vi "Write to File.vi"(8 "error in (no error)":errorcluster, 10 "INI Ref":T1, 11 "Keyboard Macro in":refnum<class "Keyboard Macro.lvclass">) -> (0 "error out":errorcluster, 2 "INI Ref out":T1, 3 "Keyboard Macro out":refnum<class "Keyboard Macro.lvclass">)   [LabVIEW 2020, in "MacroAssert.lvlib" / "Keyboard Macro.lvclass"]
uses:
  Keyboard Macro.lvclass
  Keyboard Macro.lvclass/Keyboard Macro.ctl
  Macro Step/Macro Step.lvclass
  MacroAssert.lvlib
  <vilib>/Utility/config.llb/NI_LVConfig.lvlib
  <vilib>/Utility/config.llb/Write Key (String).vi
  <vilib>/Utility/config.llb/Write Key (Boolean).vi
  <vilib>/Utility/config.llb/Config Data RefNum.ctl
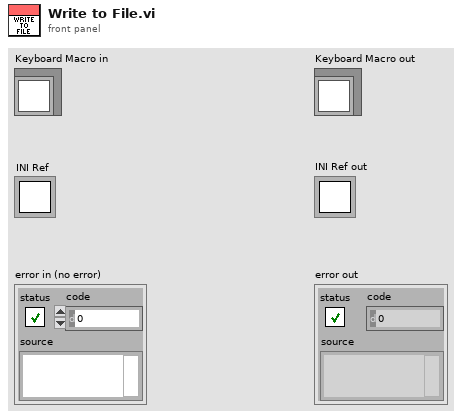
[diagram p1: front panel]
types:
  T1 = typedef "NI_LVConfig.lvlib/Config Data RefNum.ctl" = refnum<k1>
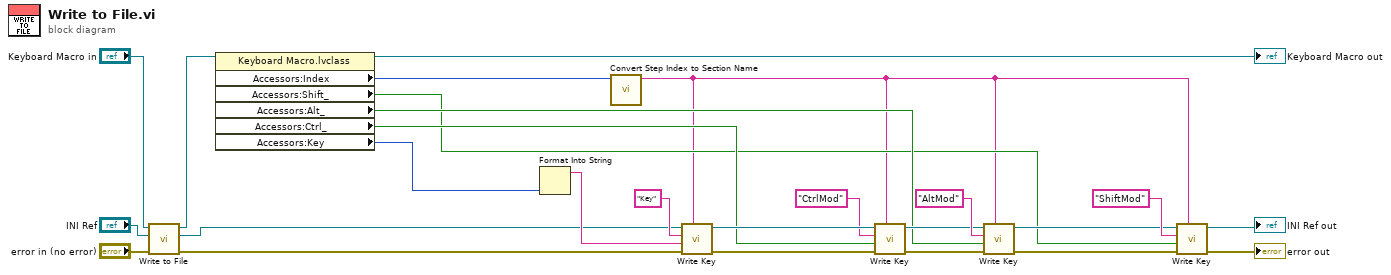
[diagram p0: block diagram]
diagram:
  n1 = call-parent "Write to File.vi"("error in (no error)"="error in (no error)", "INI Ref"="INI Ref", "Macro Step in"="Keyboard Macro in") -> ("error out"=w15:errorcluster, "INI Ref out"=w13:T1, "Macro Step out"=w14:refnum<class "Keyboard Macro.lvclass">)  [unwired: 6 in]
  n2 = property class="Keyboard Macro.lvclass"(reference=w14) -> (reference out=→"Keyboard Macro out":refnum<class "Keyboard Macro.lvclass">, "Accessors:Index"=w19:i32, "Accessors:Shift_"=w3:bool, "Accessors:Alt_"=w4:bool, "Accessors:Ctrl_"=w17:bool, "Accessors:Key"=w18:u8)  [unwired: 1 in, 1 out]
  n3 = Format Into String(w18) -> (resulting string=w16:string)  [unwired: 3 in, 1 out]
  n4 = call "Convert Step Index to Section Name.vi"("Step Index"=w19) -> ("Section Name"=w2:string)  [unwired: 10 in]
  n5 = call-poly <vilib>:"Write Key.vi"("section"=w2, "error in (no error)"=w15, "value"=w16, "key"="Key", "refnum"=w13) -> ("error out"=w21:errorcluster, "refnum out"=w23:T1)  [unwired: 4 in, 1 out]
  n6 = call-poly <vilib>:"Write Key.vi"("section"=w2, "error in (no error)"=w21, "value"=w17, "key"="CtrlMod", "refnum"=w23) -> ("error out"=w6:errorcluster, "refnum out"=w5:T1)  [unwired: 4 in, 1 out]
  n7 = call-poly <vilib>:"Write Key.vi"("section"=w2, "error in (no error)"=w6, "value"=w4, "key"="AltMod", "refnum"=w5) -> ("error out"=w10:errorcluster, "refnum out"=w8:T1)  [unwired: 4 in, 1 out]
  n8 = call-poly <vilib>:"Write Key.vi"("section"=w2, "error in (no error)"=w10, "value"=w3, "key"="ShiftMod", "refnum"=w8) -> ("error out"=→"error out":errorcluster, "refnum out"=→"INI Ref out":T1)  [unwired: 4 in, 1 out]
